vi "AdaBoostRegressor.vi"(8 "error in":errorcluster) -> (0 "error out":errorcluster, 3 "out":refnum<class "AdaBoostRegressor.lvclass">)   [LabVIEW 2020]
doc: "An AdaBoost regressor.\n\n An AdaBoost [1] regressor is a meta-estimator that begins by fitting a\n regressor on the original dataset and then fits additional copies of the\n regressor on the same dataset but where the weights of instances are\n adjusted according to the error of the current prediction. As such,\n subsequent regressors focus more on difficult cases.\n\n This class implements the algorithm known as AdaBoost.R2 [2].\n\n Read more in the :ref:`User Guide <adaboost>`.\n\n .. versionadded:: 0.14\n\n Parameters\n ----------\n base_estimator : object, default=None\n The base estimator from which the boosted ensemble is built.\n If ``None``, then the base estimator is\n :class:`~sklearn.tree.DecisionTreeRegressor` initialized with\n `max_depth=3`.\n\n n_estimators : int, default=50\n The maximum number of estimators at which boosting is terminated.\n In case of perfect fit, the learning procedure is stopped early.\n\n learning_rate : float, default=1.\n Weight applied to each classifier at each boosting iteration. A higher\n learning rate increases the contribution of each classifier. There is\n a trade-off between the `learning_rate` and `n_estimators` parameters.\n\n loss : {'linear', 'square', 'exponential'}, default='linear'\n The loss function to use when updating the weights after each\n boosting iteration.\n\n random_state : int, RandomState instance or None, default=None\n Controls the random seed given at each `base_estimator` at each\n boosting iteration.\n Thus, it is only used when `base_estimator` exposes a `random_state`.\n In addition, it controls the bootstrap of the weights used to train the\n `base_estimator` at each boosting iteration.\n Pass an int for reproducible output across multiple function calls.\n See :term:`Glossary <random_state>`.\n\n Attributes\n ----------\n base_estimator_ : estimator\n The base estimator from which the ensemble is grown.\n\n estimators_ : list of classifiers\n The collection of fitted sub-estimators.\n\n estimator_weights_ : ndarray of floats\n Weights for each estimator in the boosted ensemble.\n\n estimator_errors_ : ndarray of floats\n Regression error for each estimator in the boosted ensemble.\n\n feature_importances_ : ndarray of shape (n_features,)\n The impurity-based feature importances if supported by the\n ``base_estimator`` (when based on decision trees).\n\n Warning: impurity-based feature importances can be misleading for\n high cardinality features (many unique values). See\n :func:`sklearn.inspection.permutation_importance` as an alternative.\n\n \nAvailable methods:\nFit\nPredict\nScore\nGet Attributes\nGet Params\nSet Params"
uses:
  AdaBoostRegressor.lvclass
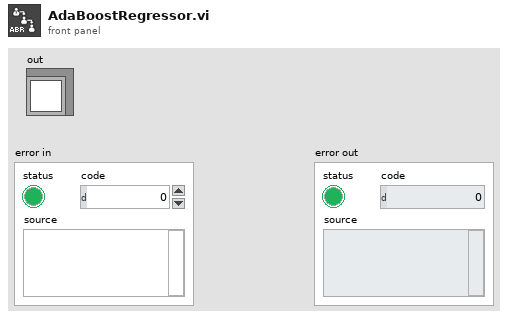
[diagram p1: front panel]
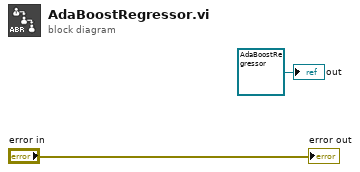
[diagram p0: block diagram]
diagram:
  "out" <- refnum<class "AdaBoostRegressor.lvclass"> refnum ("model")
  "error out" <- "error in"
